vi "Start Test.vi"(8 "error in (no error)":errorcluster, 10 "Tests":string[](array[string]), 11 "Text Report In":refnum<class "Text Report.lvclass">) -> (0 "error out":errorcluster, 3 "Text Report Out":refnum<class "Text Report.lvclass">)   [LabVIEW 2020, in "Text Report.lvclass"]
uses:
  Text Report.lvclass
  Text Report.lvclass/Text Report.ctl
  Framework/Paths/Paths.lvlib
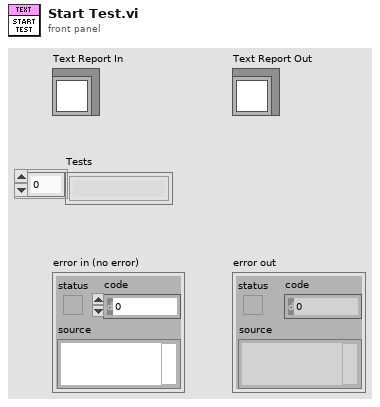
[diagram p1: front panel]
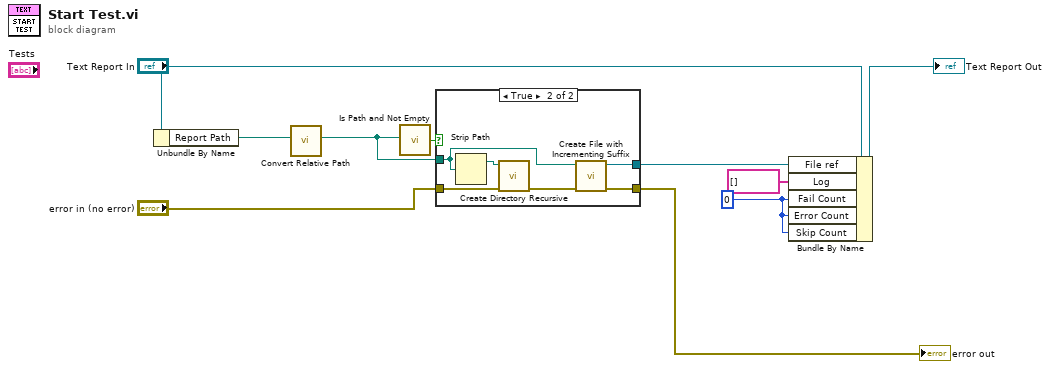
[diagram p0: block diagram]
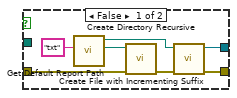
[diagram p2: hidden frame]
diagram:
  w8 = 0 ("Fail Count")
  n1 = Unbundle By Name("Text Report In") -> ("Report Path"=w2:path)
  n2 = call "Convert Relative Path.vi"("File Path in"=w2) -> ("Modified Path"=w1:path)  [unwired: 10 in]
  n3 = call <vilib>:"Is Path and Not Empty.vi"("path"=w1) -> ("Is Path and Not Empty?"=w7:bool)  [unwired: 4 in]
  n4 = case shown="True" w7 {
    tunnel: w1 -> [_ w22]
    tunnel: [w14 w23] -> w4
    tunnel: "error in (no error)" -> [w17 w19]
    tunnel: [w13 w18] -> w3
    frame False {
      n5 = call "Get Default Report Path.vi"("File Extension"="txt") -> ("Default Report Directory"=w16:path, "Default Report Path"=w12:path)  [unwired: 9 in]
      n6 = call <vilib>:"Create Directory Recursive.vi"("error in (no error)"=w17, "directory"=w16) -> ("error out"=w15:errorcluster)  [unwired: 3 in, 2 out]
      n7 = call <vilib>:"Create File with Incrementing Suffix.vi"("error in (no error)"=w15, "file path"=w12) -> ("error out"=w14:errorcluster, "refnum out"=w13:refnum<file>)  [unwired: 7 in, 1 out]
    }
    frame True {
      n8 = Strip Path(path=w22) -> (stripped path=w21:path)  [unwired: 1 out]
      n9 = call <vilib>:"Create Directory Recursive.vi"("error in (no error)"=w19, "directory"=w21) -> ("error out"=w20:errorcluster)  [unwired: 3 in, 2 out]
      n10 = call <vilib>:"Create File with Incrementing Suffix.vi"("error in (no error)"=w20, "file path"=w22) -> ("error out"=w23:errorcluster, "refnum out"=w18:refnum<file>)  [unwired: 7 in, 1 out]
    }
  }
  "error out" <- w4
  n11 = Bundle By Name(cluster="Text Report In", "File ref"=w3, "Log"=string[] [], "Fail Count"=w8, "Error Count"=w8, "Skip Count"=w8) -> (→"Text Report Out":refnum<class "Text Report.lvclass">)
